vi "Get3dPos.vi"(5 "precision (3)":i16=3, 11 "error in (no error)":errorcluster) -> (6 "(X,Y,Z) Position":string, 15 "error out":errorcluster)   [LabVIEW 2009]
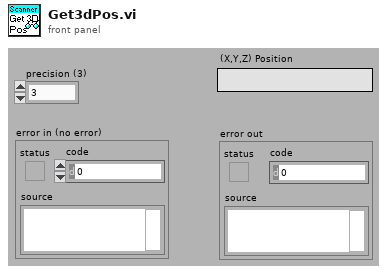
[diagram p1: front panel]
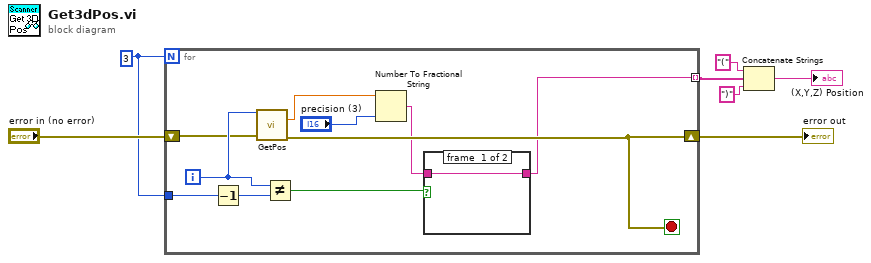
[diagram p0: block diagram]
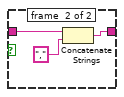
[diagram p2: hidden frame]
diagram:
  w3 = 3
  n1 = for {
    N: w3 -> [_]
    tunnel: w3 -> [w13]
    shift-right: [w12] -> w4
    shift-left: "error in (no error)" -> [w11]
    tunnel: [w8] -> w1 mode=indexing
    i -> [w15]
    stop <- w12 stop-if-true
    n2 = Decrement(x=w13) -> (x-1=w14:i32)
    n3 = call "GetPos.vi"("Axis In"=w15, "error in (no error)"=w11) -> ("Position"=w17:dbl, "error out"=w12:errorcluster)  [unwired: 10 in, 2 out]
    n4 = Not Equal?(x=w15, y=w14) -> (x != y?=w16:bool)
    n5 = Number To Fractional String(number=w17, precision (6)="precision (3)") -> (F-format string=w9:string)  [unwired: 2 in]
    n6 = case shown="True" w16 {
      tunnel: [w18 w20] -> w8
      tunnel: w9 -> [w18 w21]
      frame #0 {
      }
      frame #1 {
        n7 = Concatenate Strings(w21, "," ("string")) -> (w20:string)
      }
    }
  }
  "error out" <- w4
  n8 = Concatenate Strings("(", w1, ")" ("string")) -> (→"(X,Y,Z) Position":string)
